vi "Write session info.vi"(10 "server information":T1, 11 "basic HTTP handler dataset in":refnum<class "HTTPS handler dataset.lvclass">) -> (3 "basic HTTP handler dataset out":refnum<class "HTTPS handler dataset.lvclass">)   [LabVIEW 2016, in "HTTPS handler dataset.lvclass"]
uses:
  HTTPS handler dataset.lvclass
  HTTP server/http server info.ctl
  HTTPS handler dataset.lvclass/HTTPS handler dataset.ctl
  HTTP server/Basic HTTPS server.lvclass
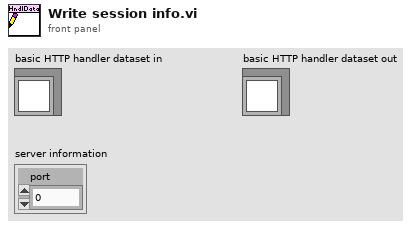
[diagram p1: front panel]
types:
  T1 = typedef "Basic HTTPS server.lvclass/http server info.ctl" = cluster{"port":u16}
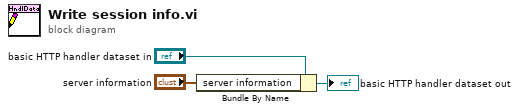
[diagram p0: block diagram]
diagram:
  n1 = Bundle By Name(cluster="basic HTTP handler dataset in", "server information"="server information") -> (→"basic HTTP handler dataset out":refnum<class "HTTPS handler dataset.lvclass">)
